vi "Read Single Sequence.vi"(6 "Segment Number (0: All segment)":i16, 8 "error in (no error)":errorcluster, 9 "Timeout (10000 ms)":u32=10000, 10 "Source (0: Channel 1)":u16(ring) items=["Channel 1", "Channel 2", "Channel 3", "Channel 4", "Memory 1", "Memory 2", "Memory 3", "Memory 4", "Function 1", "Function 2", "Function 3", "Function 4", "Function 5", "Function 6", "Function 7", "Function 8"], 11 "VISA resource name":refnum<visa-resource-name>) -> (0 "error out":errorcluster, 2 "Waveform Data":waveform(dbl)(graph), 3 "VISA resource name out":refnum<visa-resource-name>)   [LabVIEW 2020, in "LeCroy Wave Series.lvlib"]
doc: "Initiates an acquisition on all channels that you enabled with the <B>Configure Channel</B> VI. The VI waits for the acquisition to complete and returns the waveform for the Source channel you specified. If the oscilloscope did not complete the acquisition within the time period you specify with the Timeout parameter, the VI returns a time out error. A common cause for a timeout error is the acquisition was not triggered. For example, the trigger level is out of range of the waveform.\n\nCall the <B>Fetch Waveform</B> VI to obtain the segment of waveforms for each of the remaining enabled Source channels without initiating another acquisition.\n\nNote: \n\n(1) If your instrument does not support auto compensation for probe attenuation, you may need to adjust the scaling of the Waveform Data accordingly. This is handled automatically in the <B>Configure Channel</B> VI or can be done manually by multiplying the Waveform Data by the probe attenuation.\n\n(2) Sequence Acquisitions are not supported by WaveSurfer models."
uses:
  LeCroy Wave Series.lvlib
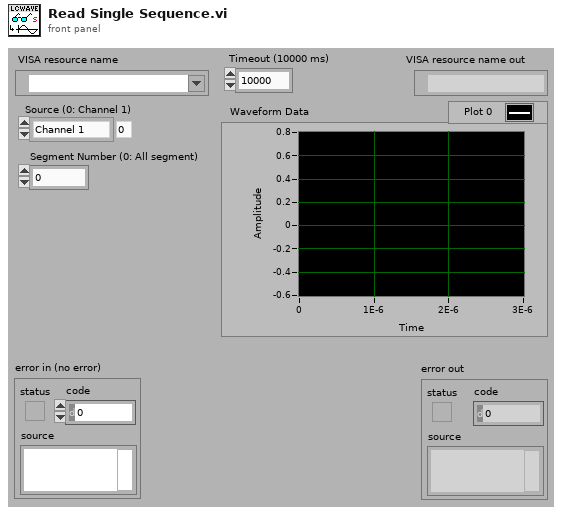
[diagram p1: front panel]
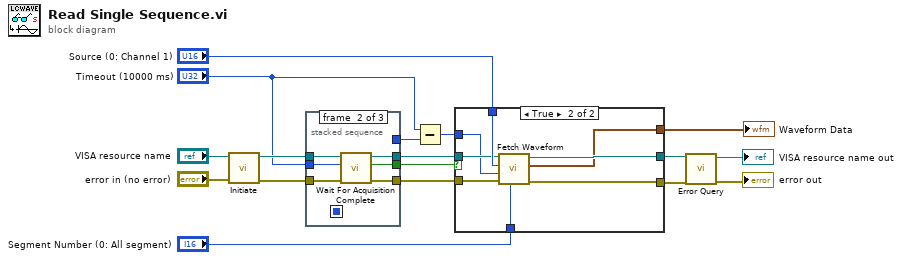
[diagram p0: block diagram]
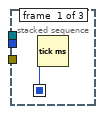
[diagram p3: hidden frame]
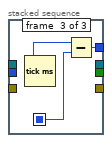
[diagram p4: hidden frame]
diagram:
  n1 = call "Initiate.vi"("error in (no error)"="error in (no error)", "VISA resource name"="VISA resource name") -> ("error out"=w11:errorcluster, "VISA resource name out"=w12:refnum<visa-resource-name>)  [unwired: 8 in]
  n2 = stacked-sequence {
    seq-local: [w18 _ _] -> [_ _ w26]
    tunnel: "Timeout (10000 ms)" -> [_ w24 _]
    tunnel: w12 -> [_ w22 _]
    tunnel: w11 -> [_ w20 _]
    tunnel: [_ w19 _] -> w7
    tunnel: [_ w21 _] -> w6
    tunnel: [_ _ w25] -> w13
    tunnel: [_ w23 _] -> w9
    frame #0 {
      n3 = Tick Count (ms)() -> (millisecond timer value=w18:u32)
    }
    frame #1 {
      n4 = call "Wait For Acquisition Complete.vi"("error in (no error)"=w20, "Timeout (10000 ms)"=w24, "VISA resource name"=w22) -> ("error out"=w19:errorcluster, "Complete"=w23:bool, "VISA resource name out"=w21:refnum<visa-resource-name>)  [unwired: 6 in]
    }
    frame #2 {
      n5 = Tick Count (ms)() -> (millisecond timer value=w27:u32)
      n6 = Subtract(x=w27, y=w26) -> (x-y=w25:u32)
    }
  }
  n7 = Subtract(x="Timeout (10000 ms)", y=w13) -> (x-y=w8:u32)
  n8 = case shown="True" w9 {
    tunnel: "Segment Number (0: All segment)" -> [_ w37]
    tunnel: "Source (0: Channel 1)" -> [_ w36]
    tunnel: w8 -> [_ w30]
    tunnel: w7 -> [w28 w35]
    tunnel: w6 -> [w29 w34]
    tunnel: [w29 w33] -> w4
    tunnel: [w28 w32] -> w3
    tunnel: [_ w31] -> w5
    frame False {
    }
    frame True {
      n9 = call "Fetch Waveform.vi"("Segment number (0: All segment)"=w37, "error in (no error)"=w35, "Timeout (10000 ms)"=w30, "Source (0: Channel 1)"=w36, "VISA resource name"=w34) -> ("error out"=w32:errorcluster, "Waveform Graph"=w31:waveform(dbl), "VISA resource name out"=w33:refnum<visa-resource-name>)  [unwired: 4 in]
    }
  }
  "Waveform Data" <- w5
  n10 = call "Error Query.vi"("error in (no error)"=w3, "VISA resource name"=w4) -> ("error out"=→"error out":errorcluster, "VISA resource name out"=→"VISA resource name out":refnum<visa-resource-name>)  [unwired: 6 in, 2 out]
